vi "AlliGator Load SS2 FLI Dataset Information.vi"(8 "error in (no error)":errorcluster, 11 "Image Folder":path) -> (0 "error out":errorcluster, 1 "Data Description":string, 2 "Metadata":string, 3 "FLI Data File Information":T1)   [LabVIEW 2021, in "AlliGator Files.lvlib"]
doc: "Loads SS2 dataset information."
uses:
  AlliGator Files.lvlib
  HDF5/AlliGator FLI Data File Information.ctl
  Phasor/Phasor Fluorescence Lifetime Parameters v3.ctl
  AlliGator FLI Dataset Type.ctl
  SwissSPAD/SS2 Extended Dataset Information.ctl
  SwissSPAD/SS2 File Information.ctl
  SwissSPAD/SS2 FPGA Parameters.ctl
  SwissSPAD/SS2 DAQ Parameters.ctl
  SwissSPAD/SS2 Data Information.ctl
  SwissSPAD/SwissSPAD 8-bit Frames Read.ctl
  SwissSPAD/SS2 HDF5 Data Blocks.ctl
  AlliGator Load Single Gate Image from SS2 Dataset.vi
  HDF5/AlliGator HDF5.lvlib
  Time/Time.lvlib
  SwissSPAD/SwissSPAD.lvlib
  <vilib>/addons/h5labview2/file/H5F.lvlib
  <vilib>/addons/h5labview2/group/H5G.lvlib
  Phasor/Phasor.lvlib
panel:
  out "elapsed (relative) seconds":dbl
  # "see the AlliGator License on the block diagram (Ctrl+E or Window:Show Block Diagram)"
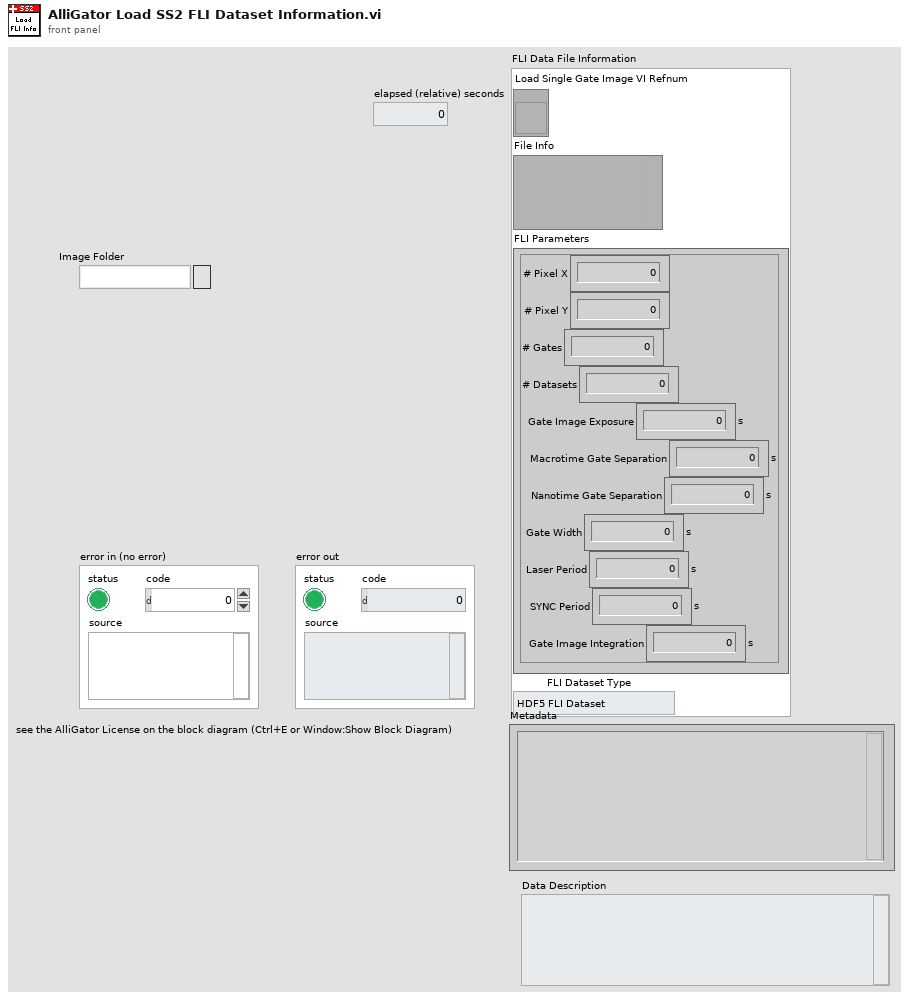
[diagram p1: front panel]
types:
  T1 = typedef "AlliGator HDF5.lvlib/AlliGator FLI Data File Information.ctl" = cluster{"Load Single Gate Image VI Refnum":refnum<vi>, "File Info":variant, "FLI Parameters":T2, "FLI Dataset Type":T3}
  T2 = typedef "Phasor.lvlib/Phasor Fluorescence Lifetime Parameters v3.ctl" = cluster{"# Pixel X":i32, "# Pixel Y":i32, "# Gates":i32, "# Datasets":i32, "Gate Image Exposure":dbl[unit], "Macrotime Gate Separation":dbl[unit], "Nanotime Gate Separation":dbl[unit], "Gate Width":dbl[unit], "Laser Period":dbl[unit], "SYNC Period":dbl[unit], "Gate Image Integration":dbl[unit]}
  T3 = typedef "AlliGator Files.lvlib/AlliGator FLI Dataset Type.ctl" = enum16{"HDF5 FLI Dataset", "Gate Image Folder", ".sdt FLI Dataset (Becker & Hickl)", ".ptu FLI Dataset (PicoQuant)", "SS1 FLI Dataset", "SS2 FLI Dataset", "I/m/phi Dataset", ".bin FLI Dataset (PicoQuant Binned)", ".bin FLI Dataset (Piccolo Binned)"}
  T4 = typedef "SwissSPAD.lvlib/SS2 Extended Dataset Information.ctl" = cluster{"File Path":path, "Swiss SPAD File Information":T5}
  T5 = typedef "SwissSPAD.lvlib/SS2 File Information.ctl" = cluster{"File Version":string, "FPGA Parameters":T6, "DAQ Parameters":T7, "Data Information":T8, "SS2 Frame Selection":T9}
  T6 = typedef "SwissSPAD.lvlib/SS2 FPGA Parameters.ctl" = cluster{"gs_no_shift":i32, "gs_no_shift_adj_1":u32, "gs_no_shift_adj_2":u32, "gs_no_shift_adj_3":u32, "gs_psincdec_0":i32, "gs_psincdec_1":u32, "gs_psincdec 2":u32, "gs_psincdec 3":u32}
  T7 = typedef "SwissSPAD.lvlib/SS2 DAQ Parameters.ctl" = cluster{"Pixel X":i32, "Pixel Y":i32, "# Gate Set":i32, "Bitness":i32, "Gate Offset":i32, "# Gate Positions":i32, "# Exposures/Frame ":i32, "Gate Step":dbl[unit], "Shutter Mode":string, "Laser Frequency":dbl[unit], "Gate Width":dbl[unit]}
  T8 = typedef "SwissSPAD.lvlib/SS2 Data Information.ctl" = cluster{"Sample Description":string, "Author":string, "Software Name":string, "Software Version":string, "Firmware Name":string, "Firmware Version":string}
  T9 = typedef "SwissSPAD.lvlib/SwissSPAD 8-bit Frames Read.ctl" = cluster{"Frame 1":bool, "Frame 2":bool, "Frame 3":bool, "Frame 4":bool}
  T10 = typedef "SwissSPAD.lvlib/SS2 HDF5 Data Blocks.ctl" = enum16{"daq_parameters", "data_information", "raw_data"}
  T11 = typedef "hid_t.ctl" = i64
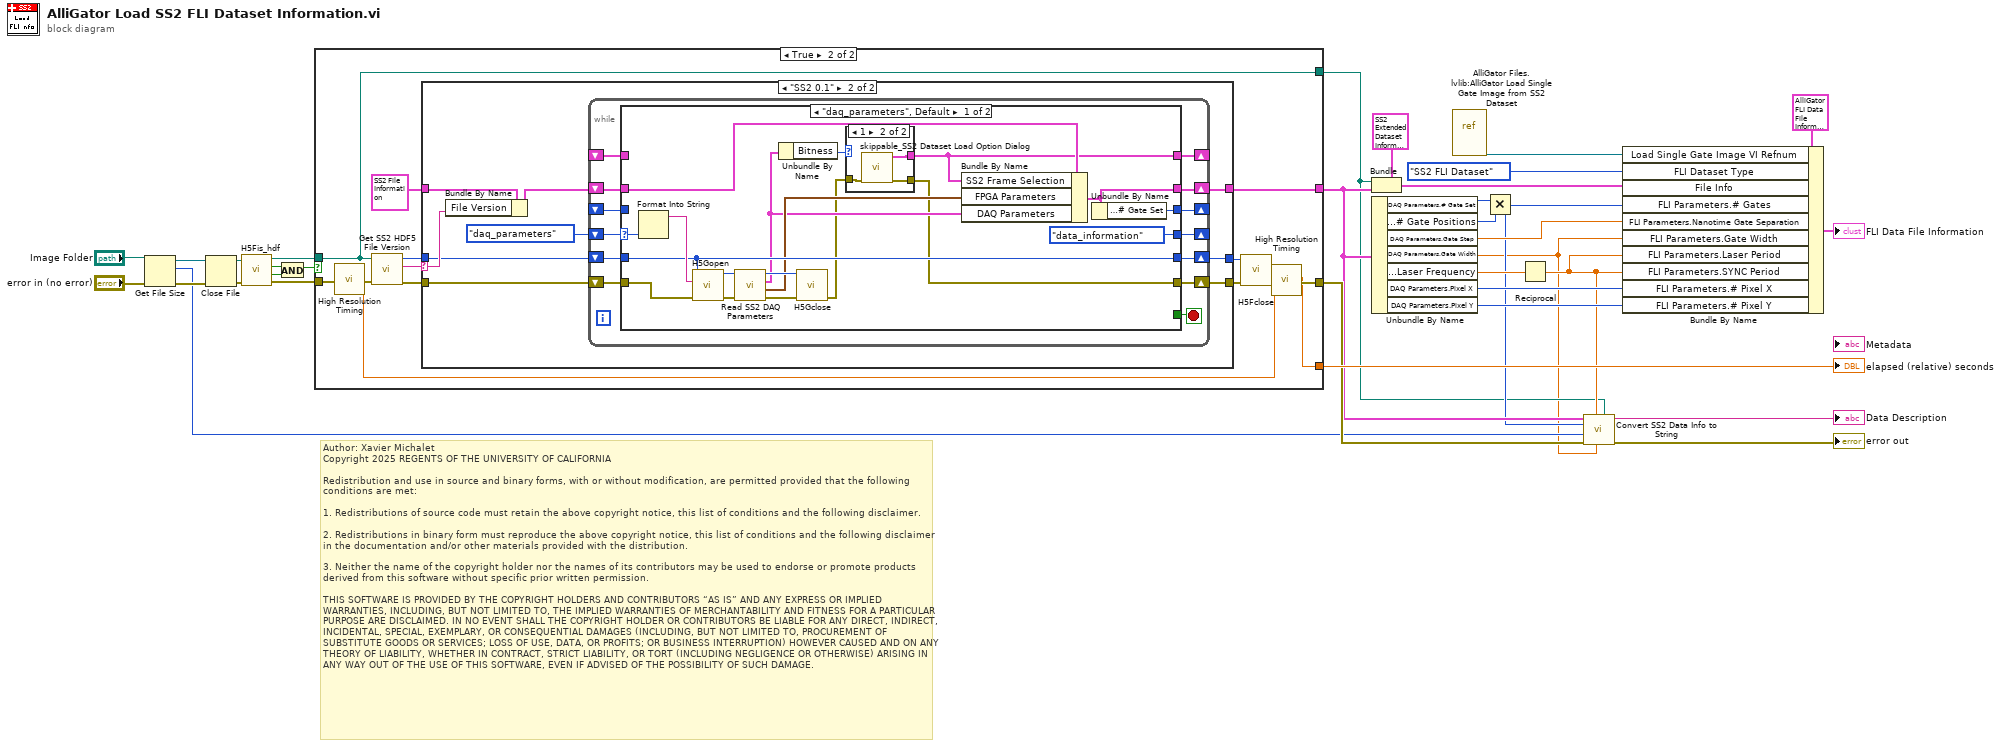
[diagram p0: block diagram]
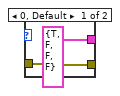
[diagram p4: hidden frame]
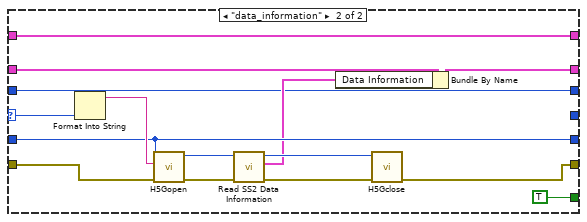
[diagram p5: hidden frame]
diagram:
  # "Author: Xavier Michalet\nCopyright 2025 REGENTS OF THE UNIVERSITY OF CALIFORNIA\n\nRedistribution and use in source and binary forms, with or without modification, are permitted provided that the following conditions are met:\n\n1. Redistributions of source code must retain the above copyright notice, this list of conditions and the following disclaimer.\n\n2. Redistributions in binary form must reproduce the above copyright notice, this list of conditions and the following disclaimer in the documentation and/or other materials provided with the distribution.\n\n3. Neither the name of the copyright holder nor the names of its contributors may be used to endorse or promote products derived from this software without specific prior written permission.\n\nTHIS SOFTWARE IS PROVIDED BY THE COPYRIGHT HOLDERS AND CONTRIBUTORS “AS IS” AND ANY EXPRESS OR IMPLIED WARRANTIES, INCLUDING, BUT NOT LIMITED TO, THE IMPLIED WARRANTIES OF MERCHANTABILITY AND FITNESS FOR A PARTICULAR PURPOSE ARE DISCLAIMED. IN NO EVENT SHALL THE COPYRIGHT HOLDER OR CONTRIBUTORS BE LIABLE FOR ANY DIRECT, INDIRECT, INCIDENTAL, SPECIAL, EXEMPLARY, OR CONSEQUENTIAL DAMAGES (INCLUDING, BUT NOT LIMITED TO, PROCUREMENT OF SUBSTITUTE GOODS OR SERVICES; LOSS OF USE, DATA, OR PROFITS; OR BUSINESS INTERRUPTION) HOWEVER CAUSED AND ON ANY THEORY OF LIABILITY, WHETHER IN CONTRACT, STRICT LIABILITY, OR TORT (INCLUDING NEGLIGENCE OR OTHERWISE) ARISING IN ANY WAY OUT OF THE USE OF THIS SOFTWARE, EVEN IF ADVISED OF THE POSSIBILITY OF SUCH DAMAGE."
  n1 = Get File Size(file="Image Folder", error in="error in (no error)") -> (refnum out=w26:refnum<file>, size (in bytes)=w6:i64, 0:w27:errorcluster)
  n2 = Close File(refnum=w26, error in=w27) -> (path=w25:path, error out=w24:errorcluster)
  n3 = call <vilib>:"H5Fis_hdf.vi"("error in (no error)"=w24, "path in"=w25) -> ("error out"=w20:errorcluster, "valid?"=w28:bool, "exists?"=w29:bool, "path out"=w21:path)  [unwired: 6 in]
  n4 = And(x=w29, y=w28) -> (x .and. y?=w19:bool)
  n5 = case shown="True" w19 {
    tunnel: w21 -> [_ w35]
    tunnel: w20 -> [w34 w36]
    tunnel: [w34 w41] -> w10
    tunnel: [_ w43] -> w7
    tunnel: [_ w39] -> w11
    tunnel: [_ w35] -> w3
    frame False {
    }
    frame True {
      n6 = call "High Resolution Timing.vi"("Error In"=w36) -> ("elapsed (relative) seconds"=w40:dbl, "Error Out"=w42:errorcluster)  [unwired: 16 in, 1 out]
      n7 = call "Get SS2 HDF5 File Version.vi"("error in (no error)"=w42, "path in"=w35) -> ("error out"=w47:errorcluster, "File Version"=w38:string, "ref out"=w37:i32)  [unwired: 7 in]
      n8 = case shown="\"SS2 0.1\"" w38 {
        selector: w38 -> [_ w53]
        tunnel: w47 -> [w51 w60]
        tunnel: [w49 w58] -> w46
        tunnel: [w51 w59] -> w45
        tunnel: T5 {"File Version"="", "FPGA Parameters"={"gs_no_shift"=0, "gs_no_shift_adj_1"=0, "gs_no_shift_adj_2"=0, "gs_no_shift_adj_3"=0, "gs_psincdec_0"=0, "gs_psincdec_1"=0, "gs_psincdec 2"=0, "gs_psincdec 3"=0}, "DAQ Parameters"={"Pixel X"=0, "Pixel Y"=0, "# Gate Set"=0, "Bitness"=0, "Gate Offset"=0, "# Gate Positions"=0, "# Exposures/Frame "=0, "Gate Step"=0.0, "Shutter Mode"="", "Laser Frequency"=0.0, "Gate Width"=0.0}, "Data Information"={"Sample Description"="", "Author"="", "Software Name"="", "Software Version"="", "Firmware Name"="", "Firmware Version"=""}, "SS2 Frame Selection"={"Frame 1"=FALSE, "Frame 2"=FALSE, "Frame 3"=FALSE, "Frame 4"=FALSE}} ("Swiss SPAD File Information") -> [w50 w55]
        tunnel: [w50 w54] -> w43
        tunnel: w37 -> [w49 w52]
        frame Default {
        }
        frame "SS2 0.1" {
          n9 = Bundle By Name(cluster=w55, "File Version"=w53) -> (w56:T5)
          n10 = while {
            shift-right: [w70] -> w59
            shift-left: w60 -> [w71]
            shift-right: [w68] -> _
            shift-left: SS2_HDF5_Data_Blocks."daq_parameters" -> [w73]
            shift-right: [w66] -> w54
            shift-left: w56 -> [w67]
            shift-right: [w65] -> _
            shift-left: _ -> [w64]
            shift-right: [w63] -> _
            shift-left: _ -> [w62]
            shift-right: [w69] -> w58
            shift-left: w52 -> [w72]
            stop <- w61 stop-if-true
            n11 = case shown="\"daq_parameters\", Default" w73 {
              selector: w73 -> [w91 w111]
              tunnel: w72 -> [w86 w105]
              tunnel: w71 -> [w89 w109]
              tunnel: [w74 w106] -> w70
              tunnel: [w86 w105] -> w69
              tunnel: [SS2_HDF5_Data_Blocks."data_information" _] -> w68
              tunnel: w67 -> [w78 w102]
              tunnel: [w81 w101] -> w66
              tunnel: [w80 w99] -> w65
              tunnel: w64 -> [_ w99]
              tunnel: [w77 w98] -> w63
              tunnel: w62 -> [_ w98]
              tunnel: [_ TRUE] -> w61
              frame "daq_parameters", Default {
                n12 = Format Into String(w91) -> (resulting string=w90:string)  [unwired: 3 in, 1 out]
                n13 = call <vilib>:"H5Gopen.vi"("error in (no error)"=w89, "name"=w90, "ref in"=w86) -> ("error out"=w88:errorcluster, "group out"=w87:T11)  [unwired: 7 in]
                n14 = call "Read SS2 DAQ Parameters.vi"("error in (no error)"=w88, "group in"=w87) -> ("error out"=w84:errorcluster, "FPGA Parameters"=w82:T6, "DAQ Parameters"=w76:T7, "group out"=w83:T11)  [unwired: 6 in]
                n15 = Unbundle By Name(w76) -> ("Bitness"=w79:i32)
                n16 = call <vilib>:"H5Gclose.vi"("error in (no error)"=w84, "group in"=w83) -> ("error out"=w75:errorcluster)  [unwired: 9 in]
                n17 = case shown="1" w79 {
                  tunnel: [T9 {"Frame 1"=TRUE, "Frame 2"=FALSE, "Frame 3"=FALSE, "Frame 4"=FALSE} ("SS2 8-bit Frame Selection") w94] -> w77
                  tunnel: w75 -> [w92 w96]
                  tunnel: [w92 w95] -> w74
                  frame 0, Default {
                  }
                  frame 1 {
                    n18 = call "skippable_SS2 Dataset Load Option Dialog.vi"("Error In"=w96) -> ("Error Out"=w95:errorcluster, "SS2 8-bit Frame Selection"=w94:T9)  [unwired: 9 in]
                  }
                }
                n19 = Bundle By Name(cluster=w78, "SS2 Frame Selection"=w77, "FPGA Parameters"=w82, "DAQ Parameters"=w76) -> (w81:T5)
                n20 = Unbundle By Name(w81) -> ("DAQ Parameters.# Gate Set"=w80:i32)
              }
              frame "data_information" {
                n21 = Format Into String(w111) -> (resulting string=w110:string)  [unwired: 3 in, 1 out]
                n22 = call <vilib>:"H5Gopen.vi"("error in (no error)"=w109, "name"=w110, "ref in"=w105) -> ("error out"=w108:errorcluster, "group out"=w107:T11)  [unwired: 7 in]
                n23 = call "Read SS2 Data Information.vi"("error in (no error)"=w108, "group in"=w107) -> ("error out"=w104:errorcluster, "Data Information"=w100:T8, "group out"=w103:T11)  [unwired: 7 in]
                n24 = Bundle By Name(cluster=w102, "Data Information"=w100) -> (w101:T5)
                n25 = call <vilib>:"H5Gclose.vi"("error in (no error)"=w104, "group in"=w103) -> ("error out"=w106:errorcluster)  [unwired: 9 in]
              }
            }
          }
        }
      }
      n26 = call <vilib>:"H5Fclose.vi"("error in (no error)"=w45, "ref"=w46) -> ("error out"=w48:errorcluster)  [unwired: 9 in]
      n27 = call "High Resolution Timing.vi"("relative seconds (NaN)"=w40, "Error In"=w48) -> ("elapsed (relative) seconds"=w39:dbl, "Error Out"=w41:errorcluster)  [unwired: 15 in, 1 out]
    }
  }
  "elapsed (relative) seconds" <- w11
  n28 = Bundle(cluster=T4 {"File Path"=path "", "Swiss SPAD File Information"={"File Version"="", "FPGA Parameters"={"gs_no_shift"=0, "gs_no_shift_adj_1"=0, "gs_no_shift_adj_2"=0, "gs_no_shift_adj_3"=0, "gs_psincdec_0"=0, "gs_psincdec_1"=0, "gs_psincdec 2"=0, "gs_psincdec 3"=0}, "DAQ Parameters"={"Pixel X"=0, "Pixel Y"=0, "# Gate Set"=0, "Bitness"=0, "Gate Offset"=0, "# Gate Positions"=0, "# Exposures/Frame "=0, "Gate Step"=0.0, "Shutter Mode"="", "Laser Frequency"=0.0, "Gate Width"=0.0}, "Data Information"={"Sample Description"="", "Author"="", "Software Name"="", "Software Version"="", "Firmware Name"="", "Firmware Version"=""}, "SS2 Frame Selection"={"Frame 1"=FALSE, "Frame 2"=FALSE, "Frame 3"=FALSE, "Frame 4"=FALSE}}} ("output cluster"), "File Path"=w3, "Swiss SPAD File Information"=w7) -> (w18:T4)
  n29 = Unbundle By Name(w7) -> ("DAQ Parameters.# Gate Set"=w17:i32, "DAQ Parameters.# Gate Positions"=w16:i32, "DAQ Parameters.Gate Step"=w15:dbl[unit], "DAQ Parameters.Gate Width"=w2:dbl[unit], "DAQ Parameters.Laser Frequency"=w14:dbl[unit], "DAQ Parameters.Pixel X"=w13:i32, "DAQ Parameters.Pixel Y"=w12:i32)
  n30 = vi-ref "AlliGator Files.lvlib:AlliGator Load Single Gate Image from SS2 Dataset.vi"() -> (w30:refnum<vi>)
  n31 = Multiply(x=w17, y=w16) -> (x*y=w5:i32)
  n32 = Reciprocal(x=w14) -> (1/x=w4:dbl[unit])
  n33 = call "Convert SS2 Data Info to String.vi"("File Path"=w3, "Step Duration"=w2, "Laser Period"=w4, "error in (no error)"=w10, "size"=w6, "# Frames"=w5, "Swiss SPAD 2 File Information"=w7) -> ("Error Out"=→"error out":errorcluster, "Data Description"=→"Data Description":string)  [unwired: 3 in]
  n34 = Bundle By Name(cluster=T1 {"Load Single Gate Image VI Refnum"=refnum, "File Info"=variant, "FLI Parameters"={"# Pixel X"=0, "# Pixel Y"=0, "# Gates"=0, "# Datasets"=0, "Gate Image Exposure"=0.0, "Macrotime Gate Separation"=0.0, "Nanotime Gate Separation"=0.0, "Gate Width"=0.0, "Laser Period"=0.0, "SYNC Period"=0.0, "Gate Image Integration"=0.0}, "FLI Dataset Type"=enum."HDF5 FLI Dataset"} ("FLI Data File Information"), "Load Single Gate Image VI Refnum"=w30, "FLI Dataset Type"=AlliGator_FLI_Dataset_Type."SS2 FLI Dataset", "File Info"=w18, "FLI Parameters.# Gates"=w5, "FLI Parameters.Nanotime Gate Separation"=w15, "FLI Parameters.Gate Width"=w2, "FLI Parameters.Laser Period"=w4, "FLI Parameters.SYNC Period"=w4, "FLI Parameters.# Pixel X"=w13, "FLI Parameters.# Pixel Y"=w12) -> (→"FLI Data File Information":T1)
